vi "FPGA ParseCompass.vi"(10 "Serial Byte":u8) -> (2 "Heading":cluster{"Yaw":dbl, "Pitch":dbl, "Roll":dbl})   [LabVIEW 2009]
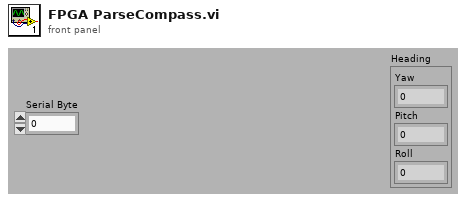
[diagram p1: front panel]
types:
  T1 = enum16{"Initialize", "Yaw", "Pitch", "Roll", "Done"}
  T2 = enum16{"Wait for $", "Check VNYPR", "skip ,", "read +-", "read numbers"}
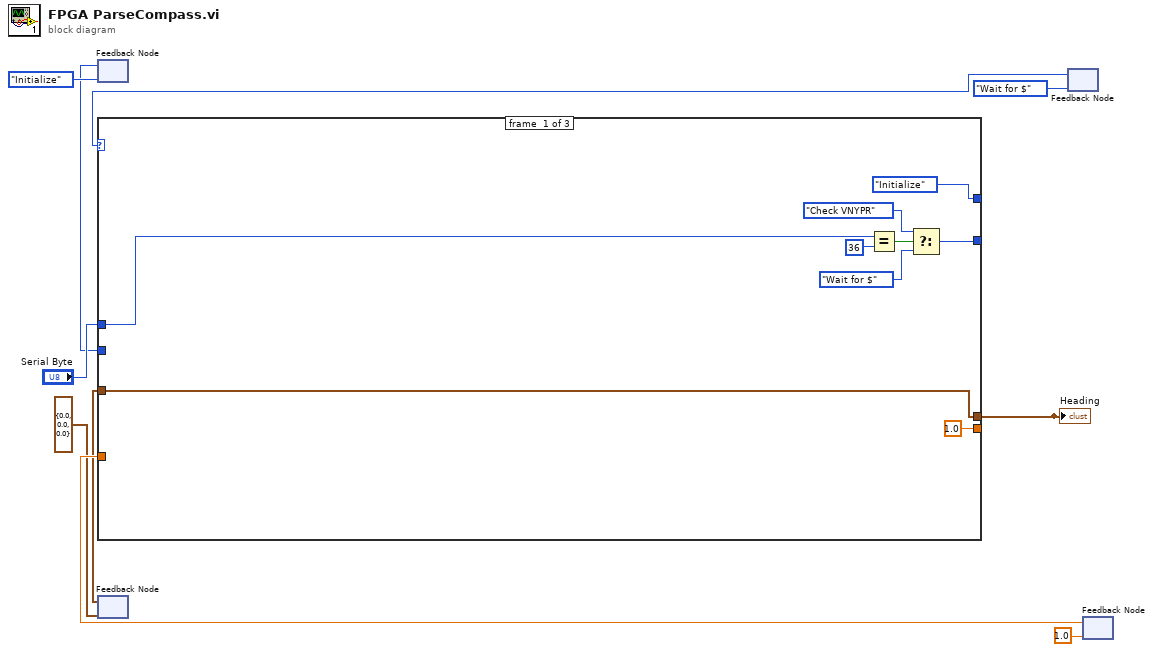
[diagram p0: block diagram]
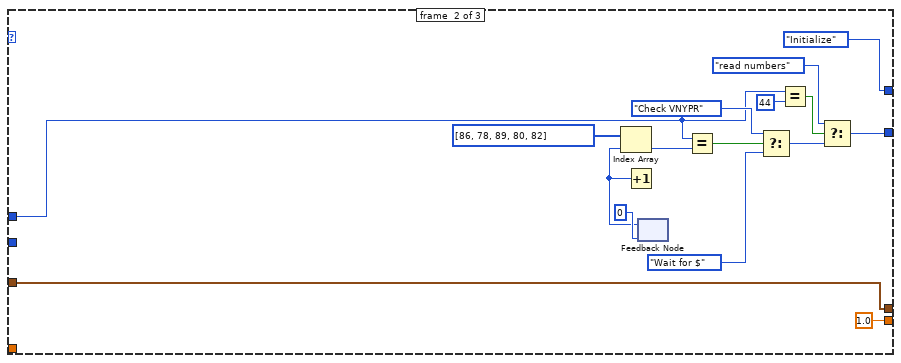
[diagram p2: hidden frame]
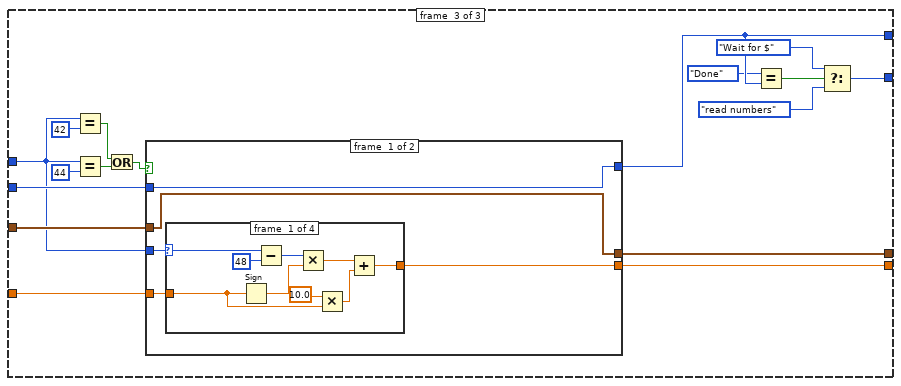
[diagram p3: hidden frame]
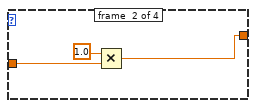
[diagram p4: hidden frame]
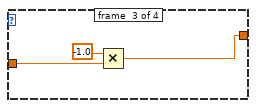
[diagram p5: hidden frame]
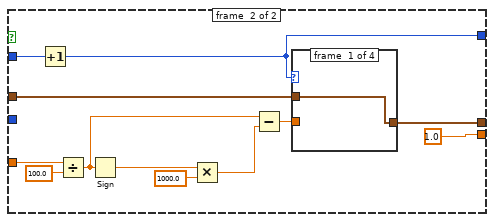
[diagram p7: hidden frame]
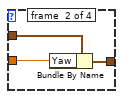
[diagram p8: hidden frame]
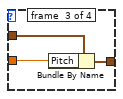
[diagram p9: hidden frame]
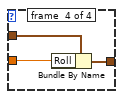
[diagram p10: hidden frame]
diagram:
  n1 = feedback #1(T1."Initialize" ("f")) -> (w1:T1)
  n2 = feedback #2(cluster{"Yaw":dbl, "Pitch":dbl, "Roll":dbl} {"Yaw"=0.0, "Pitch"=0.0, "Roll"=0.0} ("Heading")) -> (w4:cluster{"Yaw":dbl, "Pitch":dbl, "Roll":dbl})
  n3 = feedback #3(T2."Wait for $" ("f")) -> (w10:T2)
  n4 = feedback #4(1.0 ("Yaw")) -> (w8:dbl)
  n5 = case shown="\"Check VNYPR\"" w10 {
    tunnel: [w17 w25 w42] -> w13
    tunnel: "Serial Byte" -> [w22 w29 w40]
    tunnel: w8 -> [_ _ w43]
    tunnel: [1.0 ("Yaw") 1.0 ("Yaw") w44] -> w9
    tunnel: [w15 w30 w54] -> w5
    tunnel: w4 -> [w15 w30 w55]
    tunnel: [T1."Initialize" ("f") T1."Initialize" ("f") w52] -> w2
    tunnel: w1 -> [_ _ w53]
    frame #0 {
      n6 = Equal?(x=w22, y=u8 36) -> (x = y?=w20:bool)
      n7 = Select(t=T2."Check VNYPR" ("f"), s=w20, f=T2."Wait for $") -> (s? t:f=w17:T2)
    }
    frame #1 {
      n8 = feedback #5(u8 0 ("Serial Byte")) -> (w33:u8)
      n9 = Index Array(array=u8[] [86, 78, 89, 80, 82], index=w33) -> (element=w37:u8)
      n10 = Increment(x=w33) -> (x+1=w32:u8)
      n11 = Equal?(x=w29, y=w37) -> (x = y?=w34:bool)
      n12 = Select(t=T2."Check VNYPR" ("f"), s=w34, f=T2."Wait for $") -> (s? t:f=w27:T2)
      n13 = Equal?(x=w29, y=u8 44) -> (x = y?=w26:bool)
      n14 = Select(t=T2."read numbers", s=w26, f=w27) -> (s? t:f=w25:T2)
    }
    frame #2 {
      n15 = Equal?(x=w40, y=u8 42) -> (x = y?=w46:bool)
      n16 = Equal?(x=w40, y=u8 44) -> (x = y?=w47:bool)
      n17 = Or(x=w46, y=w47) -> (x .or. y?=w45:bool)
      n18 = case shown="True" w45 {
        tunnel: w55 -> [w61 w89]
        tunnel: [w61 w88] -> w54
        tunnel: [w60 w86] -> w52
        tunnel: w53 -> [w60 w87]
        tunnel: [w57 1.0 ("Yaw")] -> w44
        tunnel: w43 -> [w58 w84]
        tunnel: w40 -> [w59 _]
        frame #0 {
          n19 = case shown="46" w59 {
            selector: w59 -> [w67 _ _ _]
            tunnel: w58 -> [w68 w73 w75 w77]
            tunnel: [w62 w71 w74 w77] -> w57
            frame #0 {
              n20 = Sign(1:w68) -> (0:w64:dbl)
              n21 = Subtract(x=w67, y=u8 48) -> (x-y=w65:u8)
              n22 = Multiply(x=w65, y=w64) -> (x*y=w63:dbl)
              n23 = Multiply(x=10.0 ("Yaw"), y=w68) -> (x*y=w69:dbl)
              n24 = Add(x=w63, y=w69) -> (x+y=w62:dbl)
            }
            frame #1 {
              n25 = Multiply(x=1.0, y=w73) -> (x*y=w71:dbl)
            }
            frame #2 {
              n26 = Multiply(x=-1.0, y=w75) -> (x*y=w74:dbl)
            }
            frame #3 {
            }
          }
        }
        frame #1 {
          n27 = Increment(x=w87) -> (x+1=w86:T1)
          n28 = Divide(x=w84, y=100.0) -> (x/y=w81:dbl)
          n29 = Sign(1:w81) -> (0:w78:dbl)
          n30 = Multiply(x=w78, y=1000.0) -> (x*y=w79:dbl)
          n31 = Subtract(x=w81, y=w79) -> (x-y=w82:dbl)
          n32 = case shown="\"Yaw\"" w86 {
            tunnel: [w90 w93 w96 w99] -> w88
            tunnel: w89 -> [w90 w92 w95 w98]
            tunnel: w82 -> [_ w91 w94 w97]
            frame #0 {
            }
            frame #1 {
              n33 = Bundle By Name(cluster=w92, "Yaw"=w91) -> (w93:cluster{"Yaw":dbl, "Pitch":dbl, "Roll":dbl})
            }
            frame #2 {
              n34 = Bundle By Name(cluster=w95, "Pitch"=w94) -> (w96:cluster{"Yaw":dbl, "Pitch":dbl, "Roll":dbl})
            }
            frame #3 {
              n35 = Bundle By Name(cluster=w98, "Roll"=w97) -> (w99:cluster{"Yaw":dbl, "Pitch":dbl, "Roll":dbl})
            }
          }
        }
      }
      n36 = Equal?(x=T1."Done", y=w52) -> (x = y?=w50:bool)
      n37 = Select(t=T2."Wait for $" ("f"), s=w50, f=T2."read numbers") -> (s? t:f=w42:T2)
    }
  }
  "Heading" <- w5
